vi "PID Template Single-Channel PID.vi"(0 "process variable":i16, 1 "reset?":bool, 7 "setpoint":i16, 12 "PID gains":T1, 13 "output range":cluster{"output high":i16, "output low":i16}={"output high"=32767, "output low"=-32768}) -> (4 "output":i16)   [LabVIEW 2017]
doc: "Implements an integer PID algorithm for simple PID applications or high-speed control applications that require an efficient algorithm. The PID algorithm features control output range limiting with integrator anti-windup. The PID algorithm also features bumpless controller output for PID gain changes."
uses:
  <vilib>/Platform/TimedLoop/XDataNode/timing_clust.ctl
  <vilib>/Platform/TimedLoop/XDataNode/nitl_modes.ctl
  <vilib>/Platform/TimedLoop/XDataNode/wakeup.ctl
  <vilib>/Platform/TimedLoop/XDataNode/XDataNode.xnode
  <vilib>/Platform/TimedLoop/XDataNode/XDNodeRunTimeDep.lvlib
  <vilib>/addons/control/pid/NI_PID_FPGA.lvlib
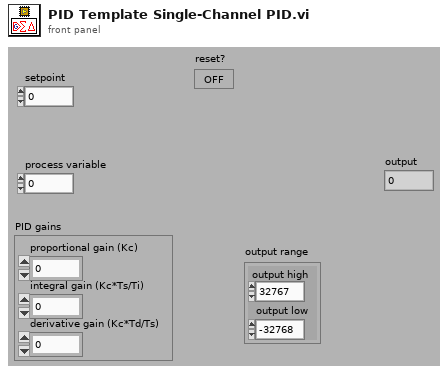
[diagram p1: front panel]
types:
  T1 = cluster{"proportional gain (Kc)":i16, "integral gain (Kc*Ts/Ti)":i16, "derivative gain (Kc*Td/Ts)":i16}
  T2 = typedef "XDNodeRunTimeDep.lvlib/timing_clust.ctl" = cluster{"Expected End [f-1]":u64, "Actual End [f-1]":u64, "Finished Late? [f-1]":bool, "Expected End [i-1]":u64, "Actual End [i-1]":u64, "Finished Late? [i-1]":bool, "Expected Start [i]":u64, "Actual Start [i]":u64, "Expected Start [f]":u64, "Actual Start [f]":u64, "Source Name":string, "Structure Name":string, "Period":i64, "Deadline":i64, "Offset":i64, "Start":i64, "Priority":i32, "Timeout":i32, "Mode":T3, "Wakeup Reason":T4, "Error":errorcluster, "Source Type":string, "Secondary Source Type":string, "Global End Time":u64, "Global Start Time":u64, "Frame Duration":u64, "Iteration Duration":u64, "Assigned CPU":i32, "I/O Scan Engine Mode":u32}
  T3 = typedef "XDNodeRunTimeDep.lvlib/nitl_modes.ctl" = enum32{"No Change", "Process missed periods, maintain original phase", "Discard missed periods, maintain original phase", "Process missed periods, ignore original phase", "Discard missed periods, ignore original phase"}
  T4 = typedef "XDNodeRunTimeDep.lvlib/wakeup.ctl" = enum32{"Normal", "Aborted", "Asynchronous wakeup", "Timing source error", "Timed loop error", "Timeout"}
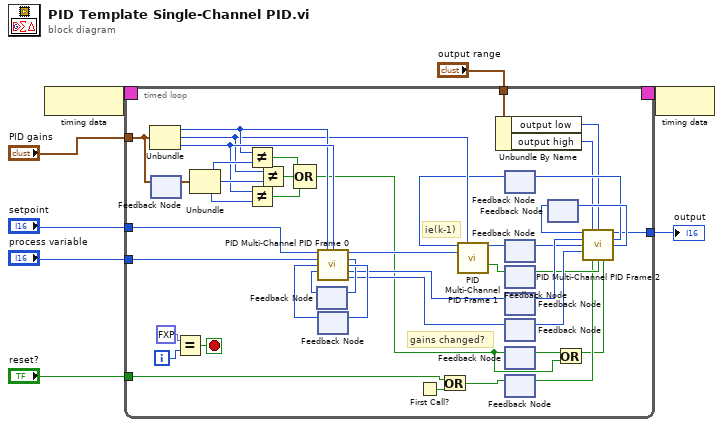
[diagram p0: block diagram]
diagram:
  n1 = node-c288() -> (w8:T2)
  n2 = timed-loop {
    timing: w8 -> [_]
    timing-out: [_] -> w7
    tunnel: "setpoint" -> [w43]
    tunnel: "process variable" -> [w42]
    tunnel: "PID gains" -> [w52]
    tunnel: "output range" -> [w26]
    tunnel: [w23] -> w2
    tunnel: "reset?" -> [w9]
    i -> [w18]
    stop <- w16 stop-if-true
    # "ie(k-1)"
    # "gains changed?"
    n3 = Unbundle(w52) -> ("proportional gain (Kc)"=w37:i16, "integral gain (Kc*Ts/Ti)"=w35:i16, "derivative gain (Kc*Td/Ts)"=w44:i16)
    n4 = feedback-in #1(w52) -> ()
    n5 = feedback #1() -> (w51:T1)  [unwired: 1 in]
    n6 = Equal?(x=fxp<+,1,1> 1.0, y=w18) -> (x = y?=w16:bool)
    n7 = Unbundle(w51) -> ("proportional gain (Kc)"=w50:i16, "integral gain (Kc*Ts/Ti)"=w48:i16, "derivative gain (Kc*Td/Ts)"=w46:i16)
    n8 = Not Equal?(x=w37, y=w50) -> (x != y?=w49:bool)
    n9 = Not Equal?(x=w44, y=w46) -> (x != y?=w45:bool)
    n10 = Not Equal?(x=w35, y=w48) -> (x != y?=w47:bool)
    n11 = Compound Arithmetic op=OR(w49, w47, w45) -> (w12:bool)
    n12 = feedback #2() -> (w39:i16)  [unwired: 1 in]
    n13 = feedback #3() -> (w40:i16)  [unwired: 1 in]
    n14 = call <vilib>:"PID Multi-Channel PID Frame 0.vi"("setpoint"=w43, "proportional gain (Kc) (k)"=w37, "derivative gain (Kc*Td/Ts) (k)"=w44, "PV(k)"=w42, "e(k-1)"=w40, "PV(k-1)"=w39) -> ("[e(k)+e(k-1)]/2"=w36:i16, "PV(k)"=w38:i16, "e(k)"=w41:i16, "u_p(k)"=w32:i32, "u_d(k)"=w31:i32)  [unwired: 5 out]
    n15 = feedback-in #2(w38) -> ()
    n16 = feedback-in #3(w41) -> ()
    n17 = First Call?() -> (First Call?: T/F=w11:bool)
    n18 = Or(x=w9, y=w11) -> (x .or. y?=w10:bool)
    n19 = Unbundle By Name(w26) -> ("output low"=w25:i16, "output high"=w24:i16)
    n20 = feedback #4() -> (w27:i32)  [unwired: 1 in]
    n21 = call <vilib>:"PID Multi-Channel PID Frame 1.vi"("ie(k-1)"=w27, "integral gain (Kc*Ts/Ti) (k)"=w35, "[e(k)+e(k-1)]/2"=w36) -> ("u_i(k)"=w30:i32, "integration off"=w29:bool)  [unwired: 11 out]
    n22 = feedback-in #5(w30) -> ()
    n23 = feedback #5() -> (w19:i32)  [unwired: 1 in]
    n24 = feedback-in #6(w29) -> ()
    n25 = feedback #6() -> (w20:bool)  [unwired: 1 in]
    n26 = feedback-in #7(w32) -> ()
    n27 = feedback #7() -> (w22:i32)  [unwired: 1 in]
    n28 = feedback-in #8(w31) -> ()
    n29 = feedback #8() -> (w21:i32)  [unwired: 1 in]
    n30 = feedback-in #9(w12) -> ()
    n31 = feedback #9() -> (w14:bool)  [unwired: 1 in]
    n32 = feedback #10() -> (w15:bool)  [unwired: 1 in]
    n33 = feedback-in #10(w10) -> ()
    n34 = feedback #11() -> (w34:i32)  [unwired: 1 in]
    n35 = Or(x=w14, y=w12) -> (x .or. y?=w13:bool)
    n36 = call <vilib>:"PID Multi-Channel PID Frame 2.vi"("output(k-1)"=w34, "output range high"=w24, "output range low"=w25, "u_p(k)"=w22, "u_i(k)"=w19, "u_d(k)"=w21, "first call or initialize?"=w15, "integration off?"=w20, "gains changed?"=w13) -> ("output"=w23:i16, "integrated effort(k)"=w28:i32, "unscaled output(k)"=w33:i32)  [unwired: 4 out]
    n37 = feedback-in #4(w28) -> ()
    n38 = feedback-in #11(w33) -> ()
  }
  "output" <- w2
  n39 = node-c288(w7) -> ()
